vi "Router - PXImc Intial Handshaking.vi"(5 "Reader Buffer Size In":u64, 6 "# Elements to Read":i32, 7 "Connection Timeout (s)":dbl, 8 "error in (no error)":errorcluster, 9 "Reader Conn ID":u16, 10 "Writer Conn ID":u16, 11 "Resource Name In":string) -> (0 "error out":errorcluster, 2 "Data Out":u32[](array[numeric]))   [LabVIEW 2016, in "PXImc Router.lvlib"]
uses:
  PXImc Router.lvlib
  <vilib>/pximc/Initialize Reader Session (U32).vi
  <vilib>/pximc/Initialize Writer Session (U32).vi
  <vilib>/pximc/Connect (U32).vi
  <vilib>/pximc/Read (U32).vi
  <vilib>/pximc/Write (U32).vi
  <vilib>/pximc/nipximc.lvlib
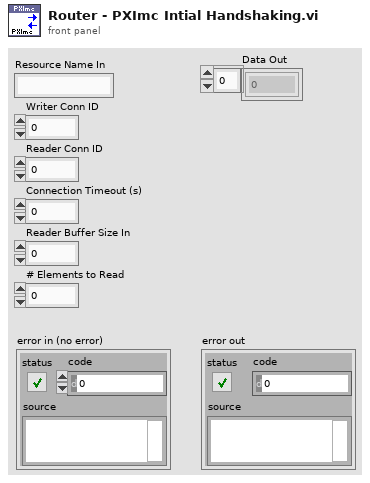
[diagram p1: front panel]
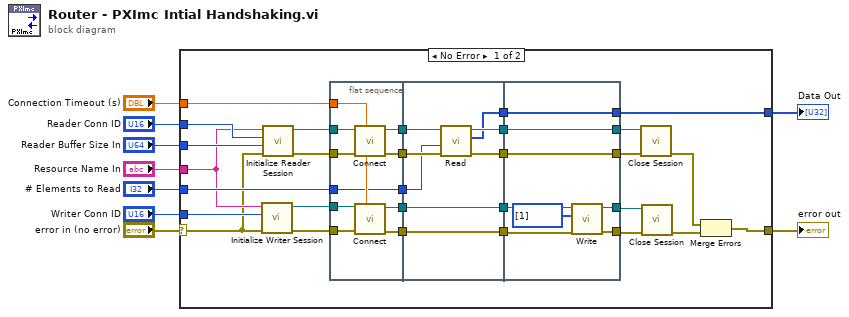
[diagram p0: block diagram]
diagram:
  n1 = case shown="No Error" "error in (no error)" {
    selector: "error in (no error)" -> [w10 w65]
    tunnel: "# Elements to Read" -> [w28 _]
    tunnel: "Reader Conn ID" -> [w27 _]
    tunnel: "Writer Conn ID" -> [w26 _]
    tunnel: "Reader Buffer Size In" -> [w25 _]
    tunnel: "Resource Name In" -> [w24 _]
    tunnel: [w23 _] -> w4
    tunnel: "Connection Timeout (s)" -> [w22 _]
    tunnel: [w17 w65] -> w2
    frame No Error {
      n2 = call-poly <vilib>:"Initialize Writer Session.vi"("error in (no error)"=w10, "connection id (1)"=w26, "interface"=w24) -> ("error out"=w14:errorcluster, "session out"=w13:refnum<k21>)  [unwired: 7 in]
      n3 = call-poly <vilib>:"Initialize Reader Session.vi"("error in (no error)"=w10, "buffer size"=w25, "writer's connection id (1)"=w27, "interface"=w24) -> ("error out"=w12:errorcluster, "session out"=w11:refnum<k21>)  [unwired: 6 in]
      n4 = flat-sequence {
        tunnel: w11 -> [w48]
        tunnel: w12 -> [w47]
        tunnel: w13 -> [w44]
        tunnel: w14 -> [w43]
        tunnel: [w46] -> w38
        tunnel: [w45] -> w37
        tunnel: [w42] -> w36
        tunnel: [w41] -> w35
        tunnel: w22 -> [w40]
        tunnel: w28 -> [w39]
        tunnel: [w39] -> w34
        tunnel: w38 -> [w54]
        tunnel: w37 -> [w52]
        tunnel: w36 -> [w56]
        tunnel: w35 -> [w55]
        tunnel: [w53] -> w33
        tunnel: [w51] -> w32
        tunnel: [w56] -> w31
        tunnel: [w55] -> w30
        tunnel: [w50] -> w29
        tunnel: w34 -> [w49]
        tunnel: [w63] -> w21
        tunnel: [w64] -> w20
        tunnel: w33 -> [w64]
        tunnel: w32 -> [w63]
        tunnel: w31 -> [w61]
        tunnel: w30 -> [w62]
        tunnel: [w60] -> w19
        tunnel: [w59] -> w18
        tunnel: w29 -> [w57]
        tunnel: [w57] -> w23
        frame #0 {
          n5 = call-poly <vilib>:"Connect.vi"("timeout in seconds (-1)"=w40, "error in (no error)"=w47, "session in"=w48) -> ("error out"=w45:errorcluster, "session out"=w46:refnum<k21>)  [unwired: 7 in]
          n6 = call-poly <vilib>:"Connect.vi"("timeout in seconds (-1)"=w40, "error in (no error)"=w43, "session in"=w44) -> ("error out"=w42:errorcluster, "session out"=w41:refnum<k21>)  [unwired: 7 in]
        }
        frame #1 {
          n7 = call-poly <vilib>:"Read.vi"("error in (no error)"=w52, "number of elements"=w49, "session in"=w54) -> ("error out"=w51:errorcluster, "data"=w50:u32[], "session out"=w53:refnum<k21>)  [unwired: 6 in]
        }
        frame #2 {
          n8 = call-poly <vilib>:"Write.vi"("error in (no error)"=w61, "data"=u32[] [1], "session in"=w62) -> ("error out"=w60:errorcluster, "session out"=w59:refnum<k21>)  [unwired: 6 in, 1 out]
        }
      }
      n9 = call <vilib>:"Close Session.vi"("error in (no error)"=w21, "session in"=w20) -> ("error out"=w15:errorcluster)  [unwired: 9 in]
      n10 = call <vilib>:"Close Session.vi"("error in (no error)"=w19, "session in"=w18) -> ("error out"=w16:errorcluster)  [unwired: 9 in]
      n11 = Merge Errors(w15, w16) -> (w17:errorcluster)
    }
    frame Error {
    }
  }
  "Data Out" <- w4
  "error out" <- w2
